vi "Max Tipper Angle.vi"() -> ()   [LabVIEW 2012]
panel:
  in  "Max Tipper Angle":dbl=1.56
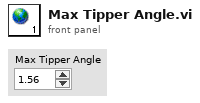
[diagram p1: front panel]
diagram:
